vi "SENS_SWE_TIME_AUTO_ON_OFF.vi"(0 "VISA IN":refnum<visa-resource-name>, 1 "Sweep Time ON/OFF":bool, 5 "error in":errorcluster, 7 "Channel":i32) -> (14 "VISA Out":refnum<visa-resource-name>, 19 "error out":errorcluster)   [LabVIEW 2018, in "PNA-X.lvlib"]
doc: "SENSe<cnum>:SWEep:TIME:AUTO <ON | OFF> \n(Read-Write) Turns the automatic sweep time function ON or OFF. \nParameters \n<cnum> Any existing channel number. If unspecified, value is set to 1 \n<ON | OFF> ON (or 1) - turns the automatic sweep time ON. \nOFF (or 0) - turns the automatic sweep time OFF. \nExamples SENS:SWE:TIME:AUTO \nsense2:sweep:time:auto off \nQuery Syntax SENSe<cnum>:SWEep:TIME:AUTO? \nReturn Type Boolean (1 = ON, 0 = OFF) \nDefault ON \n1819"
uses:
  PNA-X.lvlib
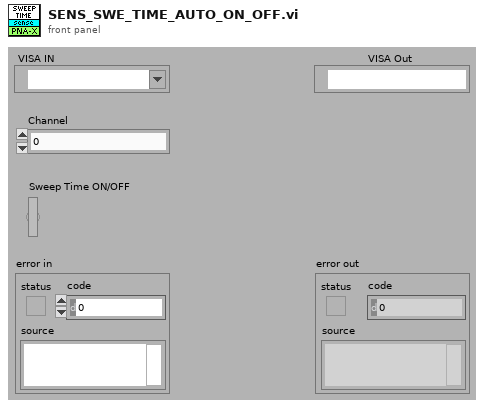
[diagram p1: front panel]
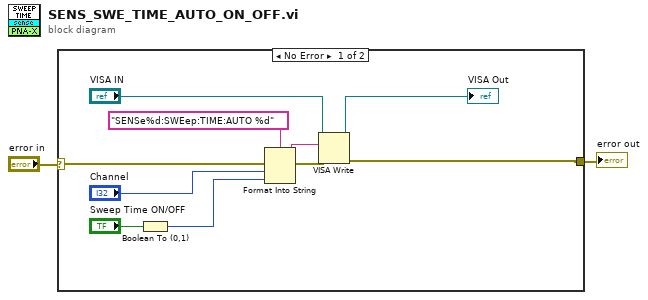
[diagram p0: block diagram]
diagram:
  n1 = case shown="No Error" "error in" {
    selector: "error in" -> [w12 w13]
    tunnel: [w7 w13] -> w1
    frame No Error {
      n2 = Boolean To (0,1)(Boolean="Sweep Time ON/OFF") -> (0, 1=w3:i16)
      n3 = Format Into String(format string="SENSe%d:SWEep:TIME:AUTO %d" ("Cmdline"), error in=w12, "Channel", w3) -> (resulting string=w10:string, error out=w11:errorcluster)  [unwired: 1 in]
      n4 = VISA Write(VISA resource name="VISA IN", write buffer=w10, error in (no error)=w11) -> (VISA resource name out=→"VISA Out":refnum<visa-resource-name>, error out=w7:errorcluster)  [unwired: 1 out]
    }
    frame Error {
    }
  }
  "error out" <- w1
